vi "ROI entry screen-Update cycle time.vi"(8 "error in (no error)":errorcluster, 10 "AXIAL MC ON ?":bool, 11 "MC ON ?":bool) -> (0 "error out":errorcluster, 1 "Cycle time (us)":dbl, 2 "Cycle time (s)":dbl, 3 "Cycle rate (Hz)":dbl)   [LabVIEW 2020]
uses:
  Typedefs/ROI management FG states.ctl
  Peripherals Control/Pockels/Globals/gl_Pockels control globals.vi
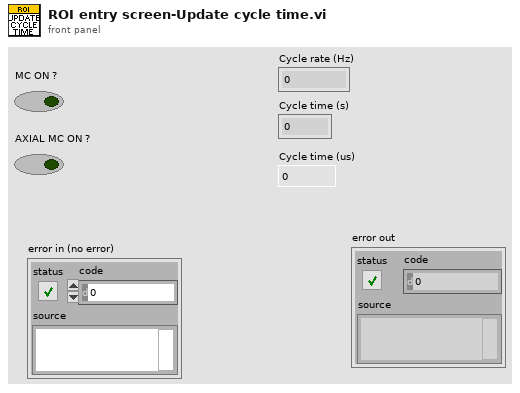
[diagram p1: front panel]
types:
  T1 = typedef "ROI management FG states.ctl" = enum16{"Read", "Write", "Write-from dataset", "Clear Last", "Clear All", "Delete ROI", "Update ROIs time", "Reload last ROI set", "Modify ROI Parameters", "Offset all ROI", "Offset visible ROI", "Modify Dwell Time", "Modify Laser Power"}
  T2 = typedef "ROI parameters data type.ctl" = cluster{"ROI index":dbl, "ROI ID":dbl, "ROI Time (ns)":dbl, "Pixels in ROI":dbl, "X start":dbl, "Y start":dbl, "Z start":dbl, "X stop":dbl, "Y stop":dbl, "Z stop":dbl, "Angle (deg)":dbl, "Composite ID":dbl, "Number of lines":dbl, "Frame Size":dbl, "Zoom":dbl, "Laser Power (%)":dbl, "ROI group ID":dbl, "Resolution":dbl, "Dwell Time per pixel":dbl, "Pixels per miniscan":dbl, "Original FOV (um)":dbl, "Apparent Frame Size":dbl, "Z Plane Idx":i32[], "Z Plane codes":i32[]}
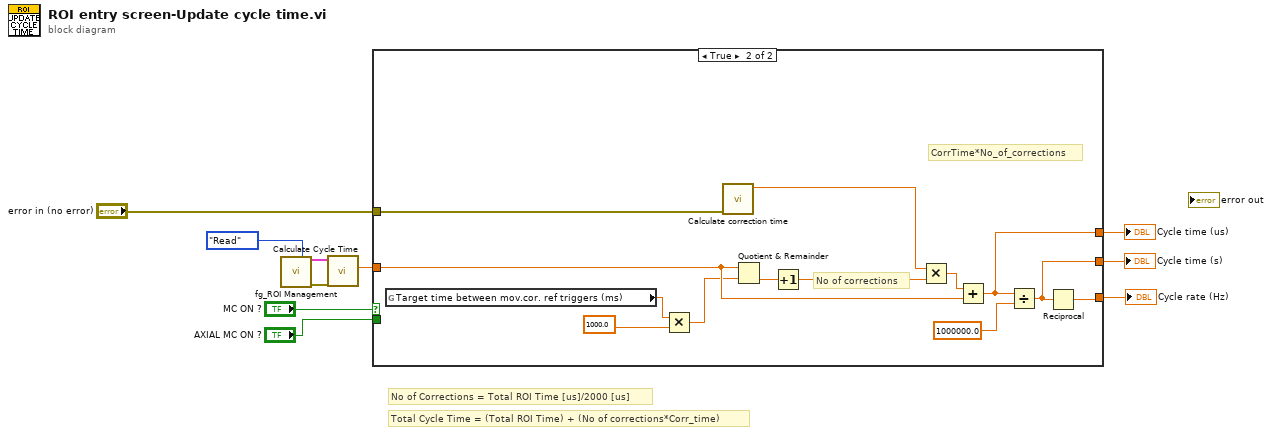
[diagram p0: block diagram]
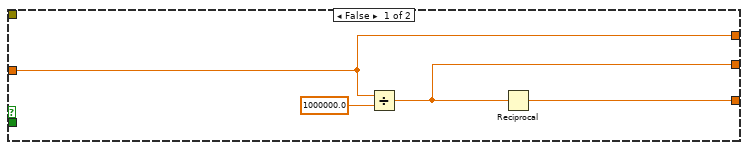
[diagram p2: hidden frame]
diagram:
  # "Total Cycle Time = (Total ROI Time) + (No of corrections*Corr_time)"
  # "No of Corrections = Total ROI Time [us]/2000 [us]"
  n1 = call "fg_ROI Management.vi"("Function"=ROI_management_FG_states."Read") -> ("ROI Setup"=w9:T2[], "error out"=w8:errorcluster)  [unwired: 8 in, 5 out]
  n2 = call "Calculate Cycle Time.vi"("error in (no error)"=w8, "Coordinates"=w9) -> ("Cycle time (us)"=w5:dbl)  [unwired: 7 in, 2 out]
  n3 = case shown="True" "MC ON ?" {
    tunnel: "AXIAL MC ON ?" -> [_ _]
    tunnel: w5 -> [w13 w25]
    tunnel: [w13 w17] -> w4
    tunnel: [w12 w22] -> w3
    tunnel: [w11 w23] -> w2
    tunnel: "error in (no error)" -> [_ w27]
    frame False {
      n4 = Divide(x=w13, y=1000000.0) -> (x/y=w12:dbl)
      n5 = Reciprocal(x=w12) -> (1/x=w11:dbl)
    }
    frame True {
      # "No of corrections"
      # "CorrTime*No_of_corrections"
      n6 = global read "gl_Pockels control globals.vi" "Target time between mov.cor. ref triggers (ms)"() -> (w16:dbl)
      n7 = Multiply(x=w16, y=1000.0) -> (x*y=w15:dbl)
      n8 = call "Calculate correction time.vi"("error in (no error)"=w27) -> ("Correction time"=w19:dbl)  [unwired: 10 in]
      n9 = Quotient & Remainder(x=w25, y=w15) -> (floor(x/y)=w21:dbl)  [unwired: 1 out]
      n10 = Increment(x=w21) -> (x+1=w20:dbl)
      n11 = Multiply(x=w19, y=w20) -> (x*y=w26:dbl)
      n12 = Add(x=w26, y=w25) -> (x+y=w17:dbl)
      n13 = Divide(x=w17, y=1000000.0) -> (x/y=w22:dbl)
      n14 = Reciprocal(x=w22) -> (1/x=w23:dbl)
    }
  }
  "Cycle time (us)" <- w4
  "Cycle time (s)" <- w3
  "Cycle rate (Hz)" <- w2
